vi "GetRectCenterPos.vi"(1 "Rect":i32[](array[numeric])) -> (0 "Cluster":cluster{dbl, dbl})   [LabVIEW 2014]
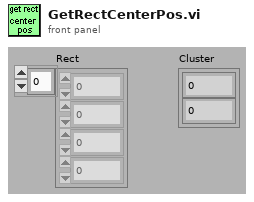
[diagram p1: front panel]
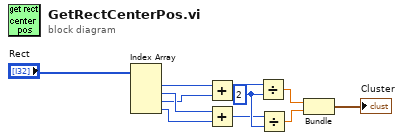
[diagram p0: block diagram]
diagram:
  w8 = 2 ("y")
  n1 = Index Array(array="Rect") -> (element #1=w2:i32, element #2=w4:i32, element #3=w3:i32, element #4=w5:i32)  [unwired: 4 in]
  n2 = Add(x=w2, y=w3) -> (x+y=w6:i32)
  n3 = Add(x=w4, y=w5) -> (x+y=w7:i32)
  n4 = Divide(x=w6, y=w8) -> (x/y=w9:dbl)
  n5 = Divide(x=w7, y=w8) -> (x/y=w10:dbl)
  n6 = Bundle(w9, w10) -> (→"Cluster":cluster{dbl, dbl})  [unwired: 1 out]
